vi "publisher tests Writer 7.vi"() -> ()   [LabVIEW 2018]
uses:
  publisher action.ctl
panel:
  out "Numeric":i32
  out "number":dbl
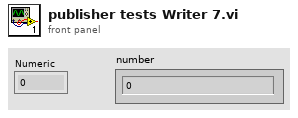
[diagram p1: front panel]
types:
  T1 = typedef "publisher action.ctl" = enum16{"set", "get", "init", "check"}
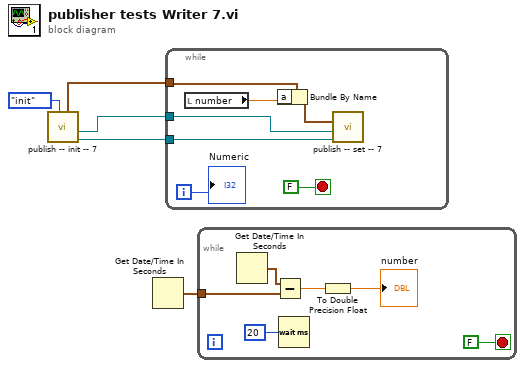
[diagram p0: block diagram]
diagram:
  n1 = call "publish -- init -- 7.vi"("publisher action"=publisher_action."init") -> ("request event"=w3:refnum<user-event>, "response ref out"=w1:refnum<vi>, "data type"=w2:cluster{"a":dbl, "b":dbl, "c":cdb})  [unwired: 8 in]
  n2 = Get Date/Time In Seconds() -> (seconds since 1Jan1904=w5:timestamp)
  n3 = while {
    tunnel: w3 -> [w10]
    tunnel: w2 -> [w9]
    tunnel: w1 -> [w6]
    i -> [w11]
    stop <- FALSE stop-if-true
    n4 = local read "number"() -> (w8:dbl)
    n5 = Bundle By Name(cluster=w9, "a"=w8) -> (w7:cluster{"a":dbl, "b":dbl, "c":cdb})
    n6 = call "publish -- set -- 7.vi"("request event"=w10, "response ref"=w6, "data"=w7) -> ()  [unwired: 9 in]
    "Numeric" <- w11
  }
  n7 = while {
    tunnel: w5 -> [w15]
    stop <- FALSE stop-if-true
    n8 = Get Date/Time In Seconds() -> (seconds since 1Jan1904=w17:timestamp)
    n9 = Subtract(x=w17, y=w15) -> (x-y=w18:dbl)
    n10 = Wait (ms)(milliseconds to wait=u32 20) -> ()  [unwired: 1 out]
    n11 = To Double Precision Float(number=w18) -> (double precision float=→"number":dbl)
  }
